vi "Check Manual.vi"(11 "Queue in":refnum<queue>) -> (3 "Manual":bool)   [LabVIEW 2014]
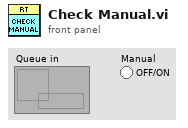
[diagram p1: front panel]
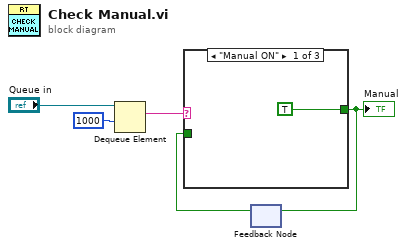
[diagram p0: block diagram]
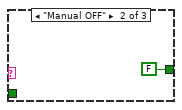
[diagram p2: hidden frame]
diagram:
  n1 = Dequeue Element(queue="Queue in", timeout in ms (-1)=1000) -> (element=w3:string)  [unwired: 1 in, 3 out]
  n2 = feedback #1() -> (w5:bool)  [unwired: 1 in]
  n3 = case shown="\"Manual ON\"" w3 {
    tunnel: [TRUE FALSE w8] -> w4
    tunnel: w5 -> [_ _ w8]
    frame "Manual ON" {
    }
    frame "Manual OFF" {
    }
    frame Default {
    }
  }
  "Manual" <- w4
  n4 = feedback-in #1(w4) -> ()
